vi "Abort.vi"(8 "error in (no error)":errorcluster, 11 "NHRDCModel in":refnum<class "NHRDCModel.lvclass">) -> (0 "error out":errorcluster, 3 "NHRDCModel out":refnum<class "NHRDCModel.lvclass">)   [LabVIEW 2018, in "AcPwrPlugins.lvlib" / "NHRDCModel.lvclass"]
uses:
  NHRDCModel.lvclass
  Database/DatabaseBaseClass/DatabaseBaseClass.lvclass
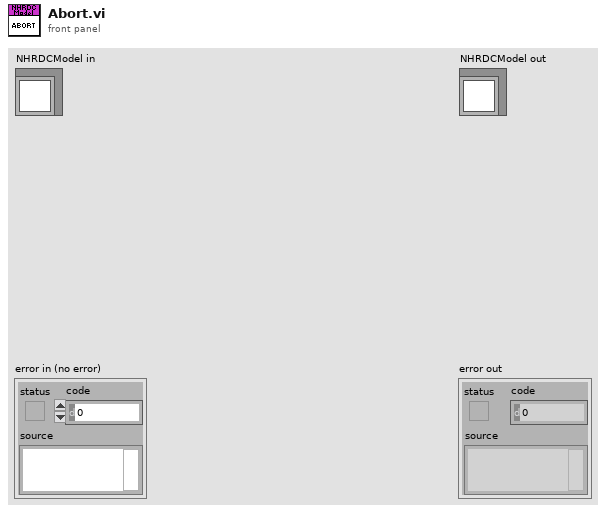
[diagram p1: front panel]
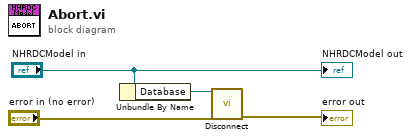
[diagram p0: block diagram]
diagram:
  n1 = Unbundle By Name("NHRDCModel in") -> ("Database"=w3:refnum<class "DatabaseBaseClass.lvclass">)
  n2 = call-dynamic "Disconnect.vi"("error in (no error)"="error in (no error)", "DatabaseBaseClass in"=w3) -> ("error out"=→"error out":errorcluster)  [unwired: 8 in, 1 out]
  "NHRDCModel out" <- "NHRDCModel in"
